vi "Create Boolean Commands.vi"(8 "Boolean States":bool[](array[boolean]), 11 "Command":string) -> (3 "Result String":string)   [LabVIEW 2014, in "Agilent MXA Series.lvlib"]
doc: "You can use this vi to create a command based on the input string and boolean states."
uses:
  Agilent MXA Series.lvlib
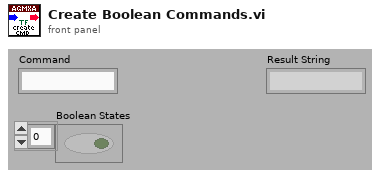
[diagram p1: front panel]
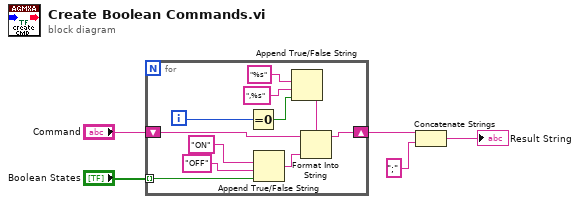
[diagram p0: block diagram]
diagram:
  n1 = for {
    shift-right: [w7] -> w3
    shift-left: "Command" -> [w8]
    tunnel: "Boolean States" -> [w6] mode=indexing
    i -> [w9]
    n2 = Equal To 0?(x=w9) -> (x = 0?=w10:bool)
    n3 = Append True/False String(1:w6, 2:"OFF" ("false string"), 3:"ON" ("true string")) -> (0:w15:string)  [unwired: 1 in]
    n4 = Append True/False String(1:w10, 2:",%s" ("format string"), 3:"%s" ("format string")) -> (0:w16:string)  [unwired: 1 in]
    n5 = Format Into String(format string=w16, initial string=w8, w15) -> (resulting string=w7:string)  [unwired: 1 in, 1 out]
  }
  n6 = Concatenate Strings(w3, ";" ("string")) -> (→"Result String":string)
